vi "Append.vi"(0 "Data":cluster{cluster{dbl, dbl}[]}[](array[cluster]), 2 "Plot":i32, 3 "X":dbl, 4 "Y":dbl) -> (14 "Data":cluster{cluster{dbl, dbl}[]}[](array[cluster]))   [LabVIEW 2018]
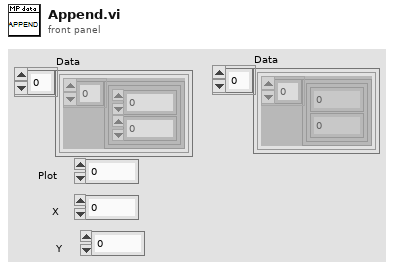
[diagram p1: front panel]
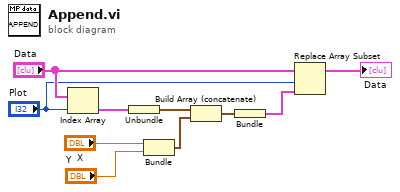
[diagram p0: block diagram]
diagram:
  n1 = Index Array(array="Data", index="Plot") -> (element=w8:cluster{cluster{dbl, dbl}[]})
  n2 = Unbundle(w8) -> (w7:cluster{dbl, dbl}[])
  n3 = Bundle("X"="X", "Y"="Y") -> (w6:cluster{"X":dbl, "Y":dbl})  [unwired: 1 in]
  n4 = Build Array (concatenate)(w7, w6) -> (w5:cluster{"X":dbl, "Y":dbl}[])
  n5 = Bundle(w5) -> (w3:cluster{cluster{"X":dbl, "Y":dbl}[]})  [unwired: 1 in]
  n6 = Replace Array Subset(array="Data", new element=w3, index="Plot") -> (→"Data":cluster{cluster{dbl, dbl}[]}[])
